vi "Set DDS Trigger Source Io.vi"(10 "io":u32, 11 "channel_index":u8) -> ()   [LabVIEW 2021, in "vmmso.lvlib"]
doc: "DLL_API void WINAPI SetDDSTriggerSourceIo(unsigned char channel_index, unsigned int io);"
uses:
  vmmso.lvlib
  vmmso.dll
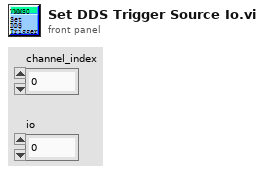
[diagram p1: front panel]
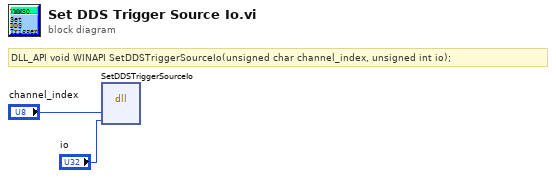
[diagram p0: block diagram]
diagram:
  # "DLL_API void WINAPI SetDDSTriggerSourceIo(unsigned char channel_index, unsigned int io);"
  n1 = dll-call lib="D:/labviewdemo/LabviewDemo 21/vmmso/vmmso.*" fn="SetDDSTriggerSourceIo"("channel_index"="channel_index", "io"="io") -> ()  [unwired: 6 in, 2 out]
